vi "2DClassificationDisplay.vi"(8 "error in":errorcluster, 11 "Parameters":T1={"Plot"=refnum, "Data"={"Split"={"X Train"=[], "X Test"=[], "Y Train"=[], "Y Test"=[]}, "Predict"=[]}, "Display"={"Choice"=enum."All", "Indexe"={"X"=0, "Y"=1}}, "Property"={"Train Style"=enum."Full circle", "Test OK Style"=enum."Full square", "Label Color"=[8978528, 4367871, 1985280], "Test NO OK"={"Style"=enum."Cross", "Color"=16716800}}}) -> (0 "error out":errorcluster)   [LabVIEW 2020]
doc: "Displays trained or tested data in 2D"
uses:
  Controls/2DParameters.ctl
  _Controls/Datas.ctl
  _Controls/PointPropertyMultipleLabel.ctl
  _Controls/Style.ctl
  _Controls/2DData.ctl
panel:
  in  "Local":T6
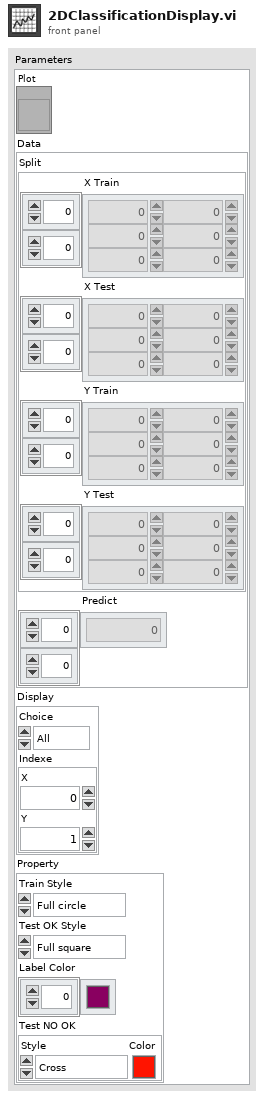
[diagram p1: front panel]
types:
  T1 = typedef "2DParameters.ctl" = cluster{"Plot":refnum<vi>, "Data":T2, "Display":cluster{"Choice":enum16{"All", "Train", "Test"}, "Indexe":cluster{"X":i32, "Y":i32}}, "Property":T3}
  T2 = typedef "Datas.ctl" = cluster{"Split":cluster{"X Train":dbl[][], "X Test":dbl[][], "Y Train":dbl[][], "Y Test":dbl[][]}, "Predict":dbl[][]}
  T3 = typedef "PointPropertyMultipleLabel.ctl" = cluster{"Train Style":T4, "Test OK Style":T4, "Label Color":u32[], "Test NO OK":cluster{"Style":T4, "Color":u32}}
  T4 = typedef "Style.ctl" = enum16{"Empty circle", "Full circle", "Empty square", "Full square", "Cross"}
  T5 = typedef "2DData.ctl" = cluster{"Tag":i32, "X":dbl[], "Y":dbl[]}
  T6 = cluster{"Parameters":T1, "2D Array":cluster{"X":dbl[], "Y":dbl[]}[], "Rating 2D Array":T5[], "Point ID":cluster{"DataUse":enum16{"Dataset", "Train", "Test"}, "Color":u32}[], "GoodPredict":i32}
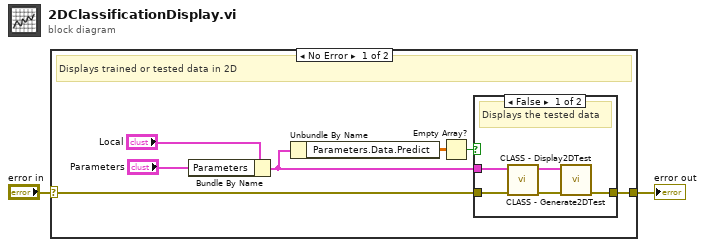
[diagram p0: block diagram]
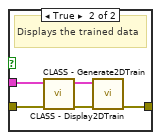
[diagram p2: hidden frame]
diagram:
  n1 = case shown="No Error" "error in" {
    selector: "error in" -> [w9 w20]
    tunnel: [w8 w20] -> w1
    frame No Error {
      # "Displays trained or tested data in 2D"
      n2 = Bundle By Name(cluster="Local", "Parameters"="Parameters") -> (w5:T6)
      n3 = Unbundle By Name(w5) -> ("Parameters.Data.Predict"=w4:dbl[][])
      n4 = Empty Array?(array=w4) -> (empty?=w3:bool)
      n5 = case shown="False" w3 {
        tunnel: w9 -> [w14 w18]
        tunnel: [w13 w19] -> w8
        tunnel: w5 -> [w10 w16]
        frame False {
          # "Displays the tested data"
          n6 = call "CLASS - Generate2DTest.vi"("error in (no error)"=w14, "Local"=w10) -> ("error out"=w12:errorcluster, "Local Out"=w11:T6)  [unwired: 8 in]
          n7 = call "CLASS - Display2DTest.vi"("error in"=w12, "Local"=w11) -> ("error out"=w13:errorcluster)  [unwired: 8 in, 1 out]
        }
        frame True {
          # "Displays the trained data"
          n8 = call "CLASS - Generate2DTrain.vi"("error in"=w18, "Local"=w16) -> ("error out"=w17:errorcluster, "Local Out"=w15:T6)  [unwired: 8 in]
          n9 = call "CLASS - Display2DTrain.vi"("error in"=w17, "Local"=w15) -> ("error out"=w19:errorcluster)  [unwired: 8 in, 1 out]
        }
      }
    }
    frame Error {
    }
  }
  "error out" <- w1
